vi "滑移力复测判定 - 副本.vi"(8 "滑移力判定项":string[][](table), 9 "压力判定项":string[][](table), 10 "拉力判定项":string[][](table), 11 "滑移力曲线":cluster{dbl[], dbl[]}[](graph)) -> (3 "判定":string[][](table))   [LabVIEW 2019]
uses:
  <vilib>/Utility/miscctls.llb/LVRowAndColumnTypeDef.ctl
  <userlib>/_MGI/1D Array/MGI Average/MGI Average (DBL[]).vi
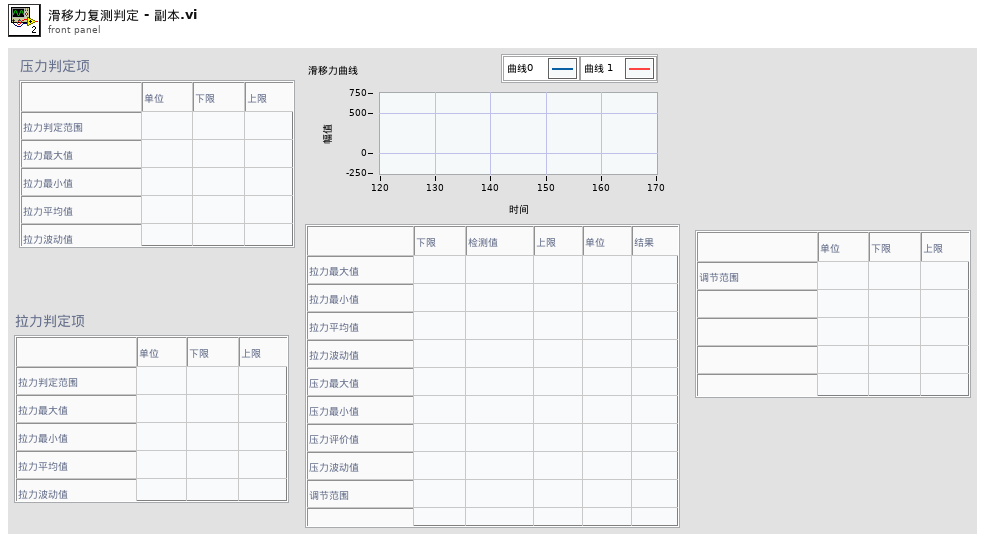
[diagram p1: front panel]
types:
  T1 = typedef "LVRowAndColumnTypeDef.ctl" = cluster{"Row":i32, "Column":i32}
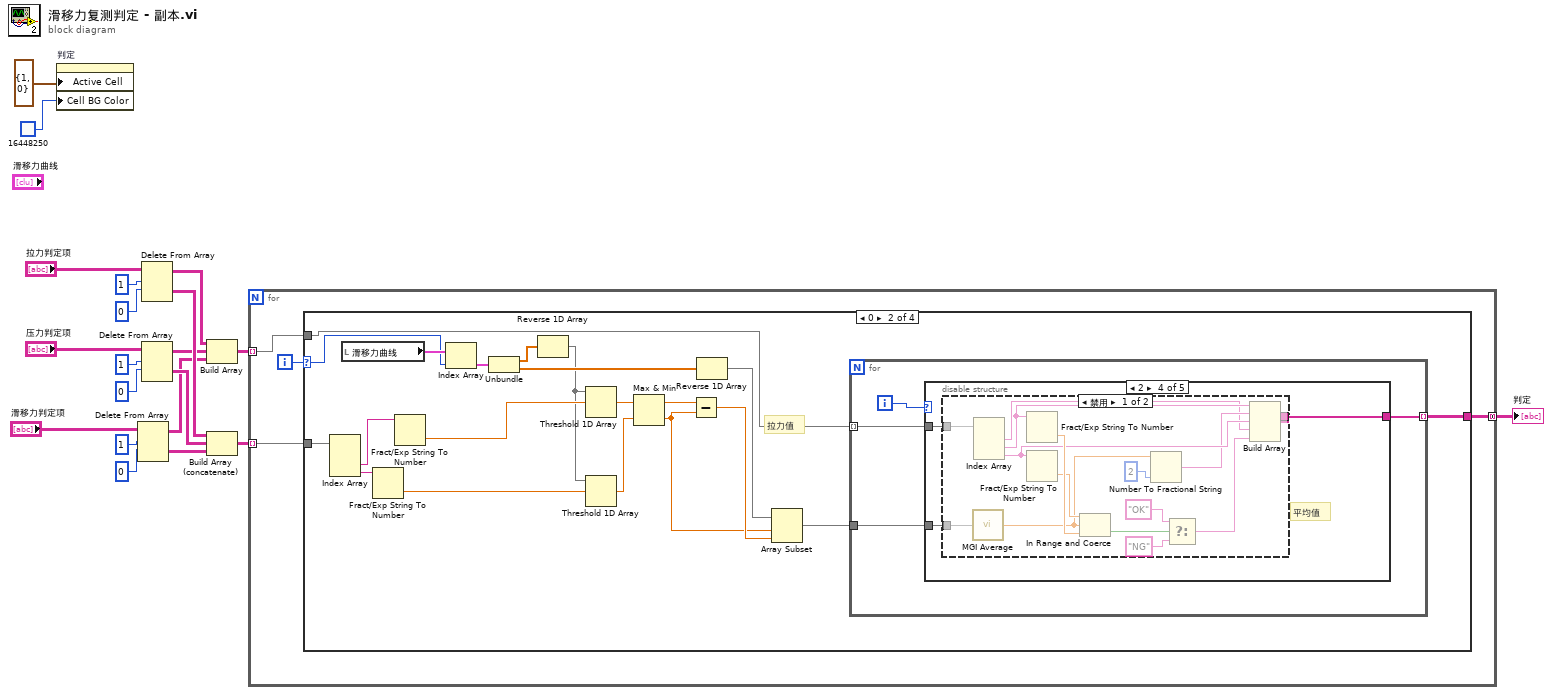
[diagram p0: block diagram]
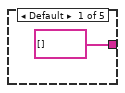
[diagram p3: hidden frame]
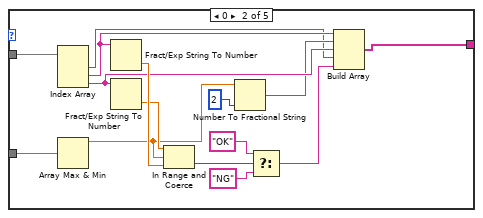
[diagram p4: hidden frame]
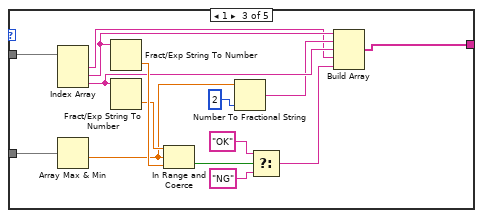
[diagram p5: hidden frame]
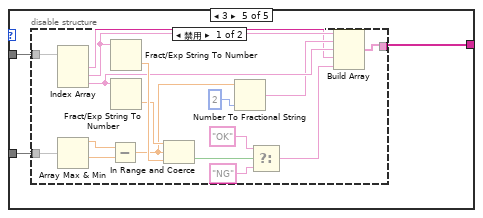
[diagram p7: hidden frame]
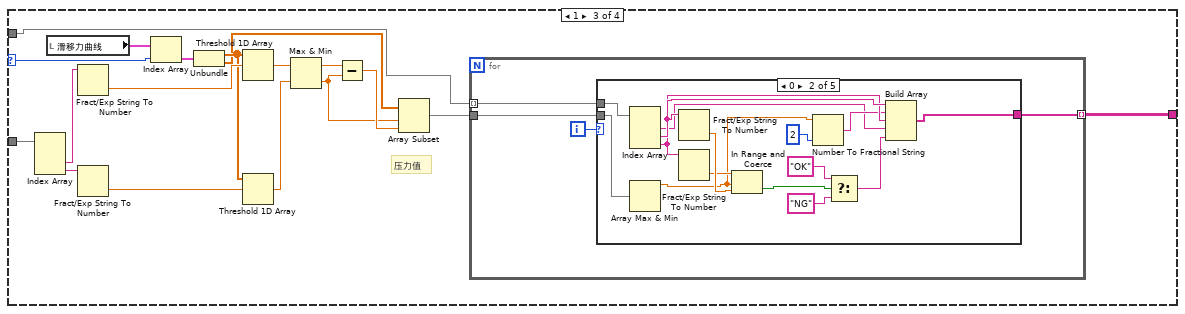
[diagram p9: hidden frame]
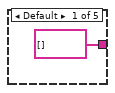
[diagram p10: hidden frame]
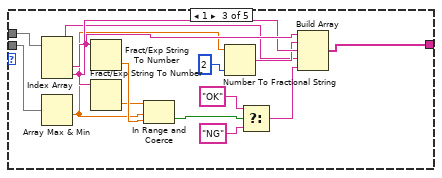
[diagram p11: hidden frame]
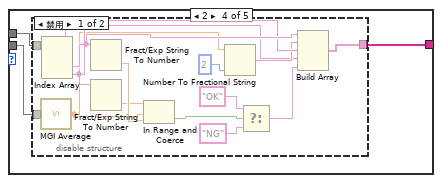
[diagram p12: hidden frame]
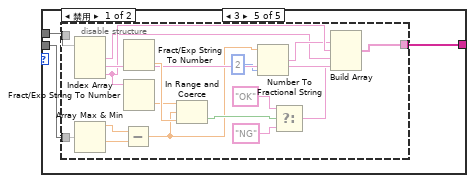
[diagram p14: hidden frame]
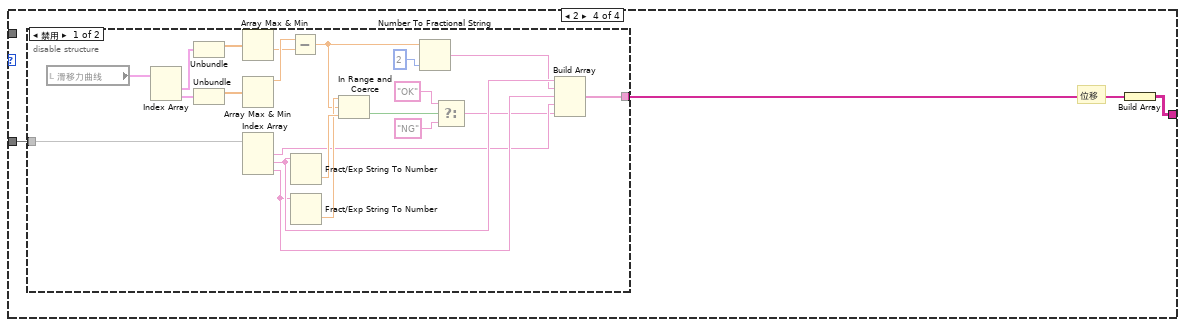
[diagram p16: hidden frame]
diagram:
  n1 = property on="判定" class="Tbl (严格)"("Active Cell"=T1 {"Row"=1, "Column"=0} ("活动单元格:活动单元格"), "Cell BG Color"=u32 16448250) -> ()  [unwired: 2 in, 2 out]
  n2 = Delete From Array(array="滑移力判定项", length=1 ("长度"), index (row)=0 ("索引 (行)")) -> (deleted portion=w4:string[][], array with subset deleted=w5:string[][])  [unwired: 1 in]
  n3 = Delete From Array(array="拉力判定项", length=1 ("长度"), index (row)=0 ("索引 (行)")) -> (deleted portion=w14:string[][], array with subset deleted=w12:string[][])  [unwired: 1 in]
  n4 = Delete From Array(array="压力判定项", length=1 ("长度"), index (row)=0 ("索引 (行)")) -> (deleted portion=w13:string[][], array with subset deleted=w11:string[][])  [unwired: 1 in]
  n5 = Build Array(w12, w11, w5) -> (w1:string[][][])
  n6 = Build Array (concatenate)(w14, w13, w4) -> (w10:string[][])
  n7 = for {
    tunnel: w10 -> [w23] mode=indexing
    tunnel: w1 -> [w22] mode=indexing
    tunnel: [w21] -> w9 mode=concatenating
    i -> [w24]
    n8 = case shown="0" w24 {
      selector: w24 -> [_ w29 w120 _]
      tunnel: w23 -> [_ w40 w133 w211]
      tunnel: w22 -> [_ w34 w125 _]
      tunnel: [_ w30 w121 w209] -> w21
      frame Default {
      }
      frame 0 {
        # "拉力值"
        n9 = Index Array(array=w40) -> (element #2=w39:string, element #3=w38:string)  [unwired: 3 in, 1 out]
        n10 = local read "滑移力曲线"() -> (w44:cluster{dbl[], dbl[]}[])
        n11 = Fract/Exp String To Number ("分数/指数字符串至数值转换")(string=w38) -> (number=w36:dbl)  [unwired: 3 in, 1 out]
        n12 = Fract/Exp String To Number(string=w39) -> (number=w37:dbl)  [unwired: 3 in, 1 out]
        n13 = Index Array(array=w44, index=w29) -> (element=w43:cluster{dbl[], dbl[]})
        n14 = Unbundle(w43) -> (w42:dbl[], w41:dbl[])
        n15 = Reverse 1D Array(array=w42) -> (reversed array=w35:dbl[])
        n16 = Threshold 1D Array ("以阈值插值一维数组")(2:w37, 3:w35) -> (0:w26:dbl)  [unwired: 1 in]
        n17 = Threshold 1D Array(2:w36, 3:w35) -> (0:w25:dbl)  [unwired: 1 in]
        n18 = Max & Min(x=w26, y=w25) -> (max(x,y)=w28:dbl, min(x,y)=w27:dbl)
        n19 = Subtract(x=w28, y=w27) -> (x-y=w32:dbl)
        n20 = Reverse 1D Array(array=w41) -> (reversed array=w33:dbl[])
        n21 = Array Subset(array=w33, index=w27, length=w32) -> (w31:dbl[])
        n22 = for {
          tunnel: w34 -> [w47] mode=indexing
          tunnel: w31 -> [w46]
          tunnel: [w45] -> w30 mode=indexing
          i -> [w48]
          n23 = case shown="2" w48 {
            tunnel: w47 -> [_ w64 w79 w82 w100]
            tunnel: w46 -> [_ w61 w76 w81 w98]
            tunnel: [string[] [] w50 w66 w80 w99] -> w45
            frame Default {
            }
            frame 0 {
              n24 = Index Array(array=w64) -> (element #1=w55:string, element #2=w60:string, element #3=w59:string)  [unwired: 3 in]
              n25 = Array Max & Min(array=w61) -> (max value=w58:dbl)  [unwired: 3 out]
              n26 = Fract/Exp String To Number(string=w60) -> (number=w63:dbl)  [unwired: 3 in, 1 out]
              n27 = Fract/Exp String To Number(string=w59) -> (number=w62:dbl)  [unwired: 3 in, 1 out]
              n28 = In Range and Coerce(upper limit=w62, x=w58, lower limit=w63) -> (In Range?=w54:bool)  [unwired: 1 out]
              n29 = Number To Fractional String(number=w58, precision (6)=i16 2 ("精度(6)")) -> (F-format string=w56:string)  [unwired: 2 in]
              n30 = Select(t="OK", s=w54, f="NG") -> (s? t:f=w51:string)
              n31 = Build Array(w60, w56, w59, w55, w51) -> (w50:string[])
            }
            frame 1 {
              n32 = Index Array(array=w79) -> (element #1=w71:string, element #2=w75:string, element #3=w74:string)  [unwired: 3 in]
              n33 = Array Max & Min(array=w76) -> (min value=w65:dbl)  [unwired: 3 out]
              n34 = Fract/Exp String To Number(string=w75) -> (number=w78:dbl)  [unwired: 3 in, 1 out]
              n35 = Fract/Exp String To Number(string=w74) -> (number=w77:dbl)  [unwired: 3 in, 1 out]
              n36 = In Range and Coerce(upper limit=w77, x=w65, lower limit=w78) -> (In Range?=w70:bool)  [unwired: 1 out]
              n37 = Number To Fractional String(number=w65, precision (6)=i16 2 ("精度(6)")) -> (F-format string=w72:string)  [unwired: 2 in]
              n38 = Select(t="OK", s=w70, f="NG") -> (s? t:f=w67:string)
              n39 = Build Array(w75, w72, w74, w71, w67) -> (w66:string[])
            }
            frame 2 {
              # "平均值"
              n40 = disable-structure shown="禁用" {
                disable-tunnel: w82 -> [w97 _]
                disable-tunnel: w81 -> [w85 _]
                disable-tunnel: [w83 _] -> w80
                frame Disabled {
                  n41 = call-poly <userlib>:"MGI Average.vi"("Double[]"=w85) -> ("Average"=w84:dbl)  [unwired: 1 in]
                  n42 = Index Array(array=w97) -> (element #1=w90:string, element #2=w94:string, element #3=w93:string)  [unwired: 3 in]
                  n43 = Fract/Exp String To Number(string=w94) -> (number=w96:dbl)  [unwired: 3 in, 1 out]
                  n44 = Fract/Exp String To Number(string=w93) -> (number=w95:dbl)  [unwired: 3 in, 1 out]
                  n45 = In Range and Coerce(upper limit=w95, x=w84, lower limit=w96) -> (In Range?=w89:bool)  [unwired: 1 out]
                  n46 = Number To Fractional String(number=w84, precision (6)=i16 2 ("精度(6)")) -> (F-format string=w91:string)  [unwired: 2 in]
                  n47 = Select(t="OK", s=w89, f="NG") -> (s? t:f=w86:string)
                  n48 = Build Array(w94, w91, w93, w90, w86) -> (w83:string[])
                }
                frame Enabled {
                }
              }
            }
            frame 3 {
              n49 = disable-structure shown="禁用" {
                disable-tunnel: w100 -> [w117 _]
                disable-tunnel: [w105 _] -> w99
                disable-tunnel: w98 -> [w104 _]
                frame Disabled {
                  n50 = Index Array(array=w117) -> (element #1=w110:string, element #2=w114:string, element #3=w113:string)  [unwired: 3 in]
                  n51 = Array Max & Min(array=w104) -> (max value=w103:dbl, min value=w102:dbl)  [unwired: 2 out]
                  n52 = Subtract(x=w103, y=w102) -> (x-y=w101:dbl)
                  n53 = Fract/Exp String To Number(string=w114) -> (number=w116:dbl)  [unwired: 3 in, 1 out]
                  n54 = Fract/Exp String To Number(string=w113) -> (number=w115:dbl)  [unwired: 3 in, 1 out]
                  n55 = In Range and Coerce(upper limit=w115, x=w101, lower limit=w116) -> (In Range?=w109:bool)  [unwired: 1 out]
                  n56 = Number To Fractional String ("数值至小数字符串转换")(number=w101, precision (6)=i16 2 ("精度(6)")) -> (F-format string=w111:string)  [unwired: 2 in]
                  n57 = Select(t="OK", s=w109, f="NG") -> (s? t:f=w106:string)
                  n58 = Build Array(w114, w111, w113, w110, w106) -> (w105:string[])
                }
                frame Enabled {
                }
              }
            }
          }
        }
      }
      frame 1 {
        # "压力值"
        n59 = Index Array(array=w133) -> (element #2=w132:string, element #3=w131:string)  [unwired: 3 in, 1 out]
        n60 = local read "滑移力曲线"() -> (w135:cluster{dbl[], dbl[]}[])
        n61 = Fract/Exp String To Number(string=w132) -> (number=w130:dbl)  [unwired: 3 in, 1 out]
        n62 = Fract/Exp String To Number(string=w131) -> (number=w129:dbl)  [unwired: 3 in, 1 out]
        n63 = Index Array(array=w135, index=w120) -> (element=w134:cluster{dbl[], dbl[]})
        n64 = Unbundle(w134) -> (w128:dbl[], w124:dbl[])
        n65 = Threshold 1D Array(2:w130, 3:w128) -> (0:w127:dbl)  [unwired: 1 in]
        n66 = Threshold 1D Array(2:w129, 3:w128) -> (0:w126:dbl)  [unwired: 1 in]
        n67 = Max & Min(x=w127, y=w126) -> (max(x,y)=w119:dbl, min(x,y)=w118:dbl)
        n68 = Subtract(x=w119, y=w118) -> (x-y=w123:dbl)
        n69 = Array Subset(array=w124, index=w118, length=w123) -> (w122:dbl[])
        n70 = for {
          tunnel: w125 -> [w138] mode=indexing
          tunnel: w122 -> [w137]
          tunnel: [w136] -> w121 mode=indexing
          i -> [w139]
          n71 = case shown="0" w139 {
            tunnel: w138 -> [_ w155 w170 w173 w191]
            tunnel: w137 -> [_ w152 w167 w171 w189]
            tunnel: [string[] [] w141 w157 w172 w190] -> w136
            frame Default {
            }
            frame 0 {
              n72 = Index Array(array=w155) -> (element #1=w146:string, element #2=w151:string, element #3=w150:string)  [unwired: 3 in]
              n73 = Array Max & Min(array=w152) -> (max value=w149:dbl)  [unwired: 3 out]
              n74 = Fract/Exp String To Number(string=w151) -> (number=w154:dbl)  [unwired: 3 in, 1 out]
              n75 = Fract/Exp String To Number(string=w150) -> (number=w153:dbl)  [unwired: 3 in, 1 out]
              n76 = In Range and Coerce(upper limit=w153, x=w149, lower limit=w154) -> (In Range?=w145:bool)  [unwired: 1 out]
              n77 = Number To Fractional String(number=w149, precision (6)=i16 2 ("精度(6)")) -> (F-format string=w147:string)  [unwired: 2 in]
              n78 = Select(t="OK", s=w145, f="NG") -> (s? t:f=w142:string)
              n79 = Build Array(w151, w147, w150, w146, w142) -> (w141:string[])
            }
            frame 1 {
              n80 = Index Array(array=w170) -> (element #1=w162:string, element #2=w166:string, element #3=w165:string)  [unwired: 3 in]
              n81 = Array Max & Min(array=w167) -> (min value=w156:dbl)  [unwired: 3 out]
              n82 = Fract/Exp String To Number(string=w166) -> (number=w169:dbl)  [unwired: 3 in, 1 out]
              n83 = Fract/Exp String To Number(string=w165) -> (number=w168:dbl)  [unwired: 3 in, 1 out]
              n84 = In Range and Coerce(upper limit=w168, x=w156, lower limit=w169) -> (In Range?=w161:bool)  [unwired: 1 out]
              n85 = Number To Fractional String(number=w156, precision (6)=i16 2 ("精度(6)")) -> (F-format string=w163:string)  [unwired: 2 in]
              n86 = Select(t="OK", s=w161, f="NG") -> (s? t:f=w158:string)
              n87 = Build Array(w166, w163, w165, w162, w158) -> (w157:string[])
            }
            frame 2 {
              n88 = disable-structure shown="禁用" {
                disable-tunnel: w173 -> [w188 _]
                disable-tunnel: [w176 _] -> w172
                disable-tunnel: w171 -> [w175 _]
                frame Disabled {
                  n89 = call-poly <userlib>:"MGI Average.vi"("Double[]"=w175) -> ("Average"=w174:dbl)  [unwired: 1 in]
                  n90 = Index Array(array=w188) -> (element #1=w181:string, element #2=w185:string, element #3=w184:string)  [unwired: 3 in]
                  n91 = Fract/Exp String To Number(string=w185) -> (number=w187:dbl)  [unwired: 3 in, 1 out]
                  n92 = Fract/Exp String To Number(string=w184) -> (number=w186:dbl)  [unwired: 3 in, 1 out]
                  n93 = In Range and Coerce(upper limit=w186, x=w174, lower limit=w187) -> (In Range?=w180:bool)  [unwired: 1 out]
                  n94 = Number To Fractional String(number=w174, precision (6)=i16 2 ("精度(6)")) -> (F-format string=w182:string)  [unwired: 2 in]
                  n95 = Select(t="OK", s=w180, f="NG") -> (s? t:f=w177:string)
                  n96 = Build Array(w185, w182, w184, w181, w177) -> (w176:string[])
                }
                frame Enabled {
                }
              }
            }
            frame 3 {
              n97 = disable-structure shown="禁用" {
                disable-tunnel: w191 -> [w208 _]
                disable-tunnel: [w196 _] -> w190
                disable-tunnel: w189 -> [w195 _]
                frame Disabled {
                  n98 = Index Array(array=w208) -> (element #1=w201:string, element #2=w205:string, element #3=w204:string)  [unwired: 3 in]
                  n99 = Array Max & Min(array=w195) -> (max value=w194:dbl, min value=w193:dbl)  [unwired: 2 out]
                  n100 = Subtract(x=w194, y=w193) -> (x-y=w192:dbl)
                  n101 = Fract/Exp String To Number(string=w205) -> (number=w207:dbl)  [unwired: 3 in, 1 out]
                  n102 = Fract/Exp String To Number(string=w204) -> (number=w206:dbl)  [unwired: 3 in, 1 out]
                  n103 = In Range and Coerce(upper limit=w206, x=w192, lower limit=w207) -> (In Range?=w200:bool)  [unwired: 1 out]
                  n104 = Number To Fractional String(number=w192, precision (6)=i16 2 ("精度(6)")) -> (F-format string=w202:string)  [unwired: 2 in]
                  n105 = Select(t="OK", s=w200, f="NG") -> (s? t:f=w197:string)
                  n106 = Build Array(w205, w202, w204, w201, w197) -> (w196:string[])
                }
                frame Enabled {
                }
              }
            }
          }
        }
      }
      frame 2 {
        # "位移"
        n107 = disable-structure shown="禁用" {
          disable-tunnel: w211 -> [w225 _]
          disable-tunnel: [w212 _] -> w210
          frame Disabled {
            n108 = local read "滑移力曲线"() -> (w232:cluster{dbl[], dbl[]}[])
            n109 = Index Array(array=w232) -> (element #1=w231:cluster{dbl[], dbl[]}, element #2=w230:cluster{dbl[], dbl[]})  [unwired: 2 in]
            n110 = Unbundle(w231) -> (w229:dbl[])  [unwired: 1 out]
            n111 = Unbundle(w230) -> (w228:dbl[])  [unwired: 1 out]
            n112 = Array Max & Min(array=w229) -> (min value=w226:dbl)  [unwired: 3 out]
            n113 = Array Max & Min(array=w228) -> (max value=w227:dbl)  [unwired: 3 out]
            n114 = Index Array(array=w225) -> (element #1=w217:string, element #2=w219:string, element #3=w218:string)  [unwired: 3 in]
            n115 = Subtract(x=w227, y=w226) -> (x-y=w215:dbl)
            n116 = Fract/Exp String To Number(string=w219) -> (number=w224:dbl)  [unwired: 3 in, 1 out]
            n117 = Fract/Exp String To Number(string=w218) -> (number=w223:dbl)  [unwired: 3 in, 1 out]
            n118 = In Range and Coerce(upper limit=w223, x=w215, lower limit=w224) -> (In Range?=w222:bool)  [unwired: 1 out]
            n119 = Number To Fractional String(number=w215, precision (6)=i16 2 ("精度(6)")) -> (F-format string=w213:string)  [unwired: 2 in]
            n120 = Select(t="OK", s=w222, f="NG") -> (s? t:f=w216:string)
            n121 = Build Array(w219, w213, w218, w217, w216) -> (w212:string[])
          }
          frame Enabled {
          }
        }
        n122 = Build Array(w210) -> (w209:string[][])
      }
    }
  }
  "判定" <- w9
